vi "Too Many Characters.vi"() -> ()   [LabVIEW 2010]
doc: "This program dispalys a message to the user if the user is trying to display too many characters for the size of the Moving Message Board display. It is only possible for this error to occur in a non-scrolling message mode of operation."
panel:
  in  "OK Button":bool
  # "You are trying to display\ntoo many characters!\n\nPlease shorten your message\nand try again."
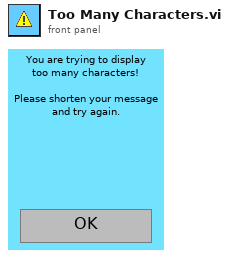
[diagram p1: front panel]
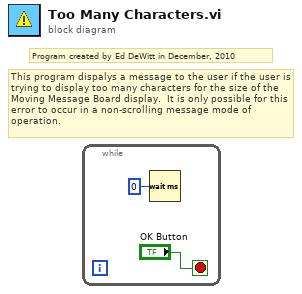
[diagram p0: block diagram]
diagram:
  # "This program dispalys a message to the user if the user is trying to display too many characters for the size of the Moving Message Board display.  It is only possible for this error to occur in a non-scrolling message mode of operation."
  # "Program created by Ed DeWitt in December, 2010"
  n1 = while {
    stop <- "OK Button" stop-if-true
    n2 = Wait (ms)(milliseconds to wait=u32 0) -> ()  [unwired: 1 out]
  }
